vi "Error - Fire Error.vi"(6 "Description":string, 8 "error in (no error)":errorcluster, 9 "Date/Time":string, 10 "Level":T1, 11 "View Model":T2) -> (0 "error out":errorcluster, 3 "View Model":T2)   [LabVIEW 2017]
doc: "Generates error user events with parameters."
uses:
  View Model/Controls/View Model.ctl
  View Model/Controls/Shared Model.ctl
  Controls/Error Model.ctl
  Controls/Error Data.ctl
  Controls/Error Level.ctl
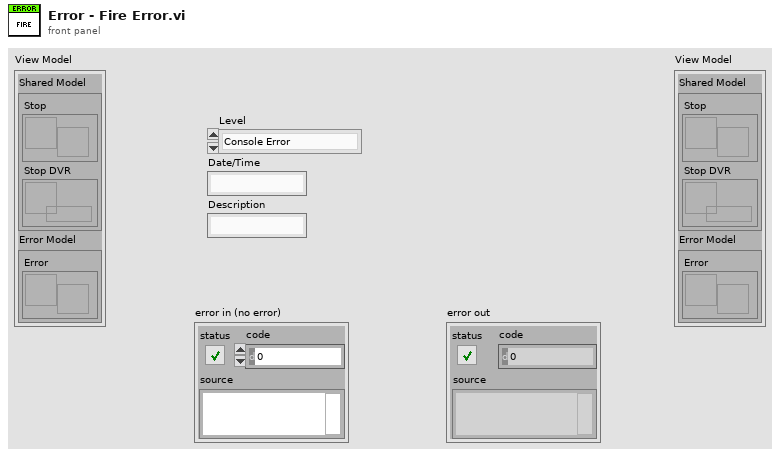
[diagram p1: front panel]
types:
  T1 = typedef "Error Level.ctl" = enum16{"Console Error", "Sensor Interface IO Error", "Process Step Error"}
  T2 = typedef "View Model.ctl" = cluster{"Shared Model":T3, "Error Model":T4}
  T3 = typedef "Shared Model.ctl" = cluster{"Stop":refnum<user-event>, "Stop DVR":refnum<data-value>}
  T4 = typedef "Error Model.ctl" = cluster{"Error":refnum<user-event>}
  T5 = typedef "Error Data.ctl" = cluster{"Level":T1, "Date/Time":string, "Description":string}
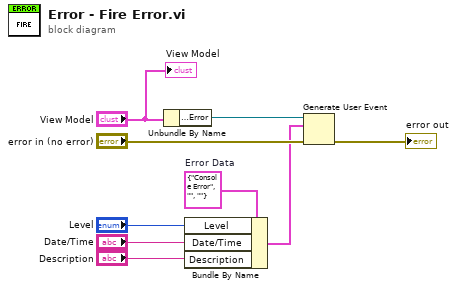
[diagram p0: block diagram]
diagram:
  w7 = T5 {"Level"=enum."Console Error", "Date/Time"="", "Description"=""}  # Error Data
  n1 = Unbundle By Name("View Model") -> ("Error Model.Error"=w9:refnum<user-event>)
  n2 = Bundle By Name(cluster=w7, "Level"="Level", "Date/Time"="Date/Time", "Description"="Description") -> (w6:T5)
  n3 = Generate User Event(user event=w9, event data cluster=w6, error in="error in (no error)") -> (error out=→"error out":errorcluster)  [unwired: 1 in, 1 out]
  "View Model" <- "View Model"
